vi "04-循环、条件结构.vi"() -> ()   [LabVIEW 2025]
panel:
  out "while计数 2":i32
  out "Boolean":bool
  out "while计数":i32
  out "Waveform Chart 2":dbl(graph)
  out "次数":i32
  out "Waveform Chart":dbl(graph)
  # "到50，灯亮\n到100，弹出“到100了”\n到150，停止循环"
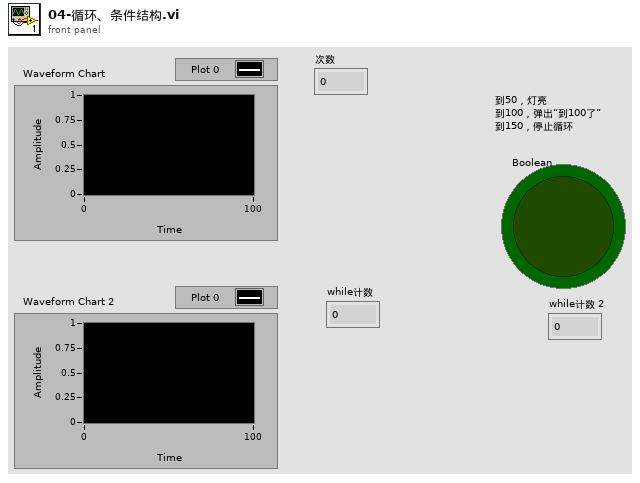
[diagram p1: front panel]
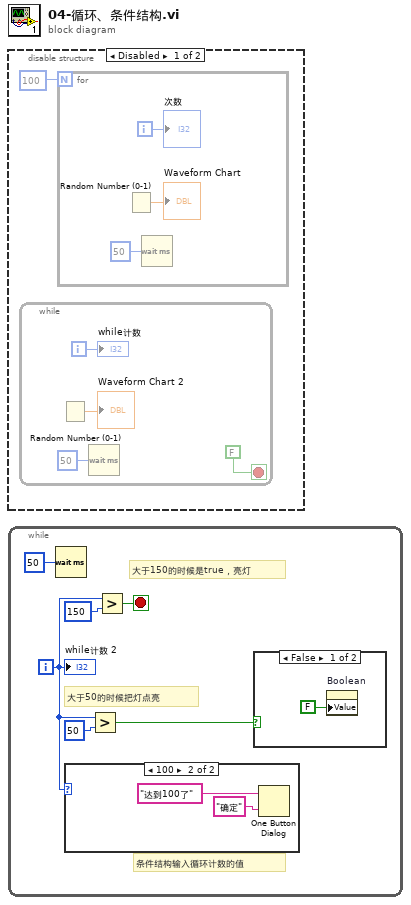
[diagram p0: block diagram]
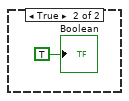
[diagram p4: hidden frame]
diagram:
  n1 = disable-structure shown="Disabled" {
    frame Disabled {
      n2 = while {
        i -> [w4]
        stop <- FALSE stop-if-true
        n3 = Random Number (0-1)() -> (number: 0 to 1=→"Waveform Chart 2":dbl)
        n4 = Wait (ms)(milliseconds to wait=u32 50) -> ()  [unwired: 1 out]
        "while计数" <- w4
      }
      n5 = for {
        N: 100 -> [_]
        i -> [w6]
        n6 = Random Number (0-1)() -> (number: 0 to 1=→"Waveform Chart":dbl)
        n7 = Wait (ms)(milliseconds to wait=u32 50) -> ()  [unwired: 1 out]
        "次数" <- w6
      }
    }
    frame Enabled {
    }
  }
  n8 = while {
    i -> [w11]
    stop <- w9 stop-if-true
    # "大于150的时候是true，亮灯"
    # "条件结构输入循环计数的值"
    # "大于50的时候把灯点亮"
    n9 = Wait (ms)(milliseconds to wait=u32 50) -> ()  [unwired: 1 out]
    n10 = case shown="100" w11 {
      frame 0, Default {
      }
      frame 100 {
        n11 = One Button Dialog(message="达到100了", button name ("OK")="确定") -> ()  [unwired: 1 out]
      }
    }
    n12 = Greater?(x=w11, y=50) -> (0:w13:bool)
    n13 = Greater?(x=w11, y=150) -> (0:w9:bool)
    n14 = case shown="False" w13 {
      frame False {
        n15 = property on="Boolean" class="Bool (strict)"("Value"=FALSE ("Boolean")) -> ()  [unwired: 2 in, 2 out]
      }
      frame True {
        "Boolean" <- TRUE ("Boolean")
      }
    }
    "while计数 2" <- w11
  }
